vi "SngJntArmSim_Execute.vi"(5 "SngJntArmSim_Model _Params":T2={"DCMOTOR_TYPES"=enum."NEO", "Num Motors"=1, "ArmLength_M"=0.75, "massKg"=26.0, "Gearing"=128.0, "MOI kgm2"=26.0, "Estimate MOI"=TRUE} {"MOI kgm2" format="%#_13g"; "Gearing" format="%#_13g"; "massKg" format="%#_13g"; "ArmLength_M" format="%#_13g"}, 7 "SngJntArmSim_Simulation _Params":T1={"MinAngle_Rad"=0.0, "MaxAngle_Rad"=0.0, "Measurment StdDev"=0.09, "SimulateGravity"=TRUE} {"Measurment StdDev" format="%#_13g"}, 8 "dT_Seconds":dbl=0.02 format="%#_13g", 9 "Battery Volts":dbl=12.0, 11 "Motor Dmd":dbl) -> (0 "Error":bool, 1 "AtLowLimit":bool, 2 "At HIgh LImit":bool, 3 "ArmAngle_Rad":dbl, 4 "Motor Current":dbl, 6 "SingleJointArmSim":T4 {"GearBox"."Jr_KgM2" format="%13.5p"; "GearBox"."L_H" format="%13.5p"; "GearBox"."Kt_NMPerAmp" format="%13.5p"; "GearBox"."KvINV_RadPerSecPerVolt" format="%13.5p"; "GearBox"."R_Ohms" format="%13.5p"; "GearBox"."FreeSpeed_RadPerSec" format="%13.5p"; "GearBox"."FreeCurrent_Amps" format="%13.5p"; "GearBox"."StallCurrent_Amps" format="%13.5p"; "GearBox"."StallTorque_NM" format="%13.5p"; "GearBox"."nominalVoltage_Volts" format="%13.5p"})   [LabVIEW 2019, in "Trajectory_Library.lvlib"]
doc: "The single jointed arm linear system definition is:\n - States\n - angle position (Rad)\n - Inputs:\n - motor voltage\n - Outputs:\n - angle position (rad)"
uses:
  Trajectory_Library.lvlib
  TypeDef/SINGLE_JOINT_ARM_SIM.ctl
  TypeDef/LINEAR_SYSTEM_SIM.ctl
  TypeDef/LINEAR_SYSTEM.ctl
  <vilib>/Analysis/Matrix/Datatypes/RealMatrix.ctl
  TypeDef/DCMOTOR.CTL
  TypeDef/LINEAR_SYSTEM_ID_SINGLE_JOINT_ARM_MODEL.ctl
  Enum/DCMOTOR_TYPES_ENUM.ctl
  TypeDef/SINGLE_JOINT_ARM_SIM_SIMULATION_PARAMS.ctl
  MatBuilder_Create.vi
  DCMotor_GetCIM.vi
  DCMotor_GetAndymark9015.vi
  DCMotor_GetAndymarkRs775_125.vi
  DCMotor_GetBag.vi
  DCMotor_GetBanebotsRs550.vi
  DCMotor_GetBanebotsRs775.vi
  DCMotor_GetFalcon500.vi
  DCMotor_GetMiniCIM.vi
  DCMotor_GetNEO.vi
  DCMotor_GetNEO550.vi
  DCMotor_GetRomiBuiltIn.vi
  DCMotor_GetVex775Pro.vi
  DCMotor_GetAndymarkAM2235A.vi
  DCMotor_GetAndymarkAM3493.vi
  DCMotor_New.vi
  Units_RotationsPerMinuteToRadiansPerSecond.vi
  <vilib>/Analysis/Matrix/NI_Matrix.lvlib
panel:
  out "Velocity_RadsPerSec":dbl
  # "<States, 1>"
  # "<Outputs, 1>"
  # "<Inputs, 1>"
  # "<Outputs, 1>"
  # "<States,States>"
  # "<States,Inputs>"
  # "<Outputs,States>"
  # "<Outputs,Inputs>"
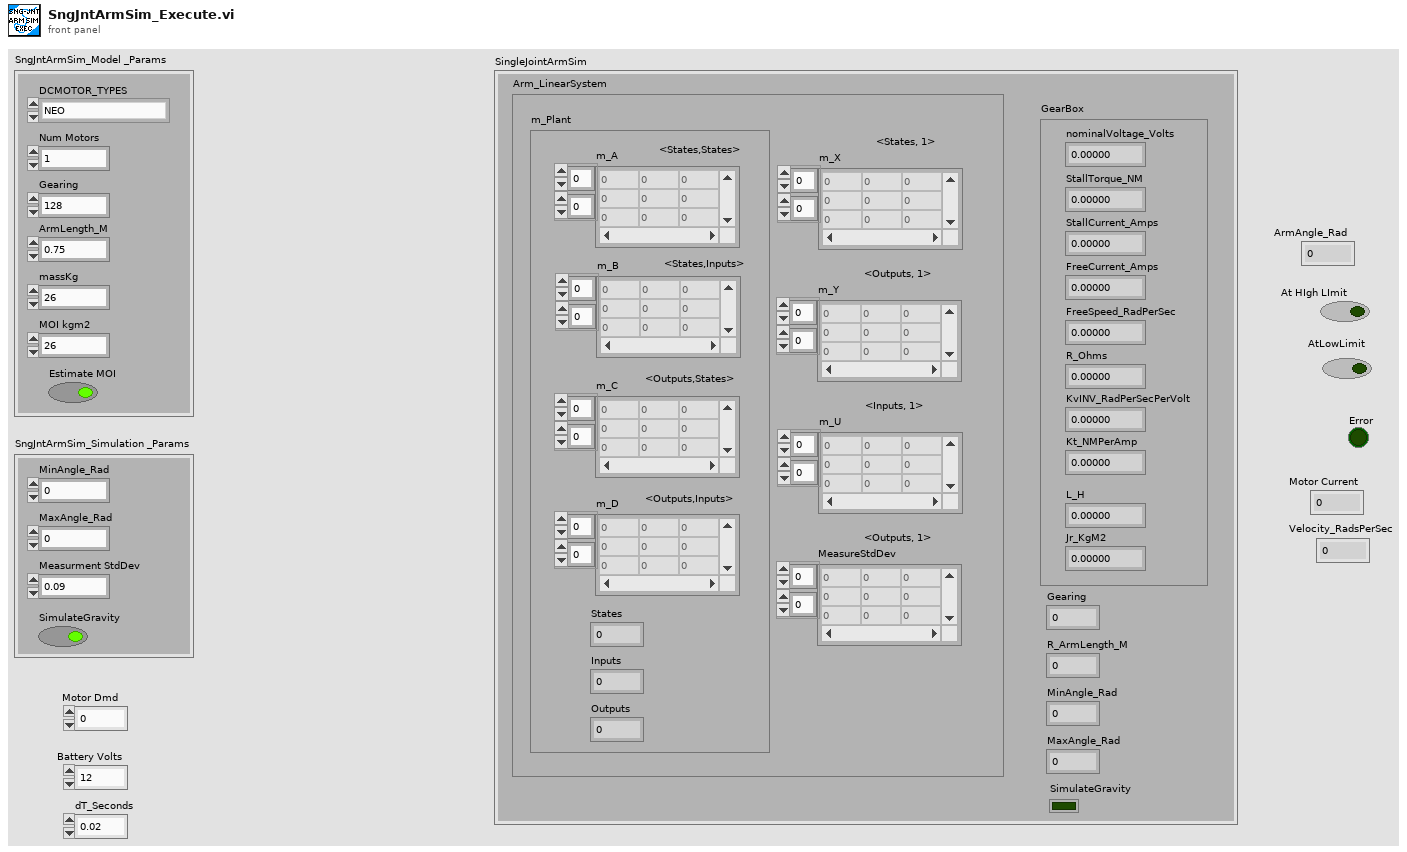
[diagram p1: front panel]
types:
  T1 = typedef "Trajectory_Library.lvlib/SINGLE_JOINT_ARM_SIM_SIMULATION_PARAMS.ctl" = cluster{"MinAngle_Rad":dbl, "MaxAngle_Rad":dbl, "Measurment StdDev":dbl, "SimulateGravity":bool}
  T2 = typedef "Trajectory_Library.lvlib/LINEAR_SYSTEM_ID_SINGLE_JOINT_ARM_MODEL.ctl" = cluster{"DCMOTOR_TYPES":T3, "Num Motors":i32, "ArmLength_M":dbl, "massKg":dbl, "Gearing":dbl, "MOI kgm2":dbl, "Estimate MOI":bool}
  T3 = typedef "Trajectory_Library.lvlib/DCMOTOR_TYPES_ENUM.ctl" = enum16{"CIM", "AndyMark 9015", "Andy Mark RS 775 125", "Bag", "BaneBots RS 550", "BaneBots RS 775", "Falcon 500", "Mini CIM", "NEO", "NEO 550", "Romi BuiltIn", "Vex 775 Pro", "Snow Blower AM 2235A", "Bosch Seat AM 3493"}
  T4 = typedef "Trajectory_Library.lvlib/SINGLE_JOINT_ARM_SIM.ctl" = cluster{"Arm_LinearSystem":T5, "GearBox":T8, "Gearing":dbl, "R_ArmLength_M":dbl, "MinAngle_Rad":dbl, "MaxAngle_Rad":dbl, "SimulateGravity":bool}
  T5 = typedef "Trajectory_Library.lvlib/LINEAR_SYSTEM_SIM.ctl" = cluster{"m_Plant":T6, "m_X":T7, "m_Y":T7, "m_U":T7, "MeasureStdDev":T7}
  T6 = typedef "Trajectory_Library.lvlib/LINEAR_SYSTEM.ctl" = cluster{"m_A":T7, "m_B":T7, "m_C":T7, "m_D":T7, "States":i32, "Inputs":i32, "Outputs":i32}
  T7 = typedef "NI_Matrix.lvlib/RealMatrix.ctl" = dbl[][]
  T8 = typedef "Trajectory_Library.lvlib/DCMOTOR.CTL" = cluster{"nominalVoltage_Volts":dbl, "StallTorque_NM":dbl, "StallCurrent_Amps":dbl, "FreeCurrent_Amps":dbl, "FreeSpeed_RadPerSec":dbl, "R_Ohms":dbl, "KvINV_RadPerSecPerVolt":dbl, "Kt_NMPerAmp":dbl, "L_H":dbl, "Jr_KgM2":dbl}
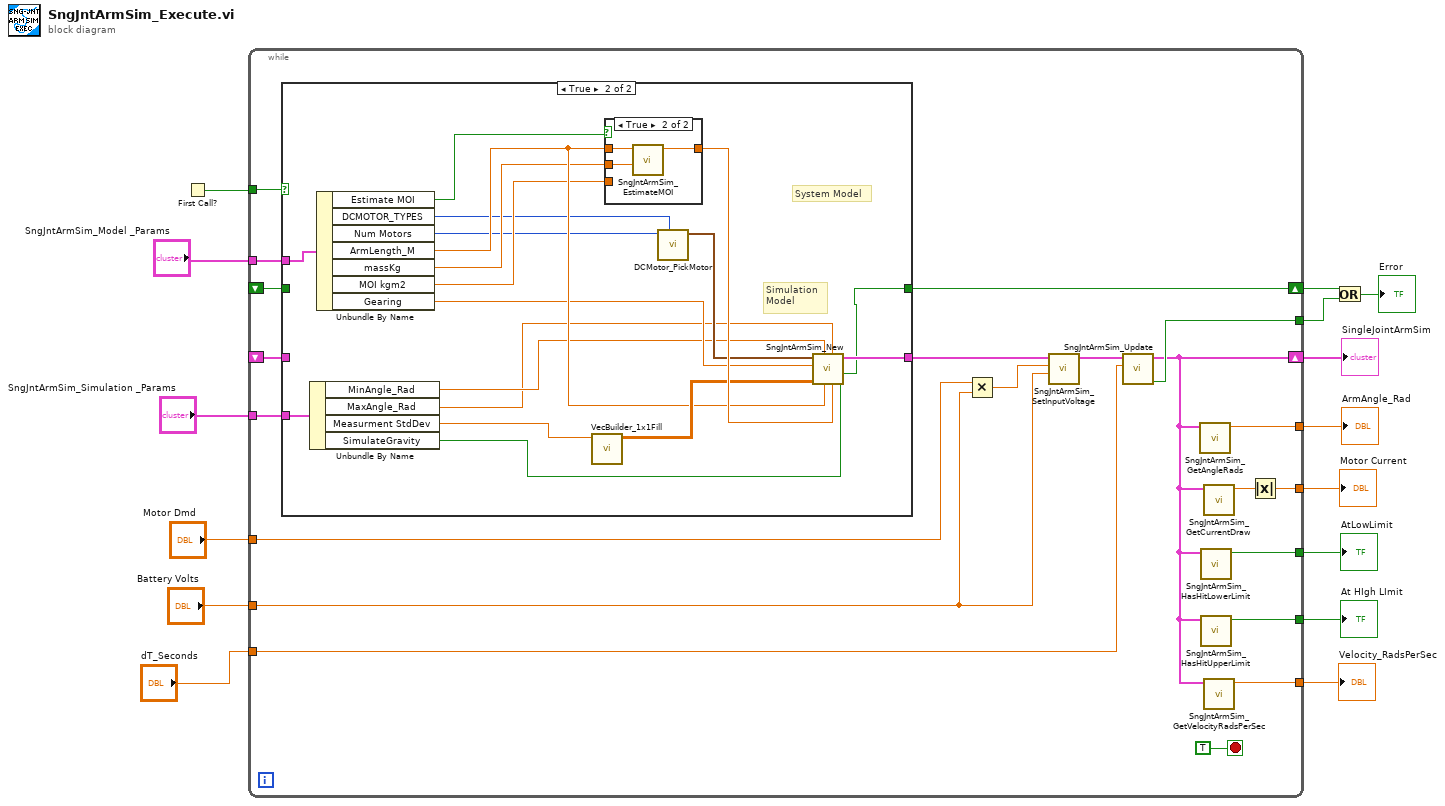
[diagram p0: block diagram]
diagram:
  n1 = First Call?() -> (First Call?: T/F=w13:bool)
  n2 = while {
    tunnel: "SngJntArmSim_Model _Params" -> [w36]
    tunnel: w13 -> [w35]
    shift-right: [w17] -> w15
    shift-left: _ -> [w34]
    shift-right: [w33] -> w6
    shift-left: _ -> [w32]
    tunnel: "Motor Dmd" -> [w27]
    tunnel: "Battery Volts" -> [w26]
    tunnel: [w25] -> w10
    tunnel: [w23] -> w9
    tunnel: [w22] -> w8
    tunnel: [w21] -> w7
    tunnel: [w20] -> w5
    tunnel: "dT_Seconds" -> [w19]
    tunnel: "SngJntArmSim_Simulation _Params" -> [w18]
    tunnel: [w16] -> w1
    stop <- TRUE stop-if-true
    n3 = case shown="True" w35 {
      tunnel: [w38 w53] -> w28
      tunnel: w36 -> [_ w52]
      tunnel: w34 -> [w38 _]
      tunnel: [w37 w39] -> w33
      tunnel: w32 -> [w37 _]
      tunnel: w18 -> [_ w44]
      frame False {
      }
      frame True {
        # "Simulation \nModel"
        # "System Model"
        n4 = Unbundle By Name(w44) -> ("MinAngle_Rad"=w41:dbl, "MaxAngle_Rad"=w40:dbl, "Measurment StdDev"=w43:dbl, "SimulateGravity"=w42:bool)
        n5 = Unbundle By Name(w52) -> ("Estimate MOI"=w45:bool, "DCMOTOR_TYPES"=w46:T3, "Num Motors"=w47:i32, "ArmLength_M"=w51:dbl, "massKg"=w48:dbl, "MOI kgm2"=w49:dbl, "Gearing"=w50:dbl)
        n6 = call "VecBuilder_1x1Fill.vi"("R0_C0"=w43) -> ("output matrix"=w55:T7)  [unwired: 10 in]
        n7 = case shown="True" w45 {
          tunnel: [w57 w60] -> w56
          tunnel: w48 -> [_ w59]
          tunnel: w51 -> [_ w58]
          tunnel: w49 -> [w57 _]
          frame False {
          }
          frame True {
            n8 = call "SngJntArmSim_EstimateMOI.vi"("ArmMass_Kg"=w59, "ArmLength_M"=w58) -> ("MOI"=w60:dbl)  [unwired: 9 in]
          }
        }
        n9 = call "DCMotor_PickMotor.vi"("DCMOTOR_TYPES"=w46, "Num Motors"=w47) -> ("DCMOTOR"=w54:T8)  [unwired: 9 in]
        n10 = call "SngJntArmSim_New.vi"("SimulateGravity"=w42, "jKgMetersSquared"=w56, "MaxAngle_Rad"=w40, "ArmLength_Meters"=w51, "MinAngle_Rad"=w41, "MeasurementStdDev"=w55, "Gearing"=w50, "GearBox"=w54) -> ("Error"=w39:bool, "SingleJointArmSim"=w53:T4)  [unwired: 2 in]
      }
    }
    n11 = Multiply(x=w27, y=w26) -> (x*y=w31:dbl)
    n12 = call "SngJntArmSim_SetInputVoltage.vi"("Battery_Volts"=w26, "Input_Voltage"=w31, "in SingleJointArmSim"=w28) -> ("out SingleJointArmSim"=w29:T4)  [unwired: 8 in]
    n13 = call "SngJntArmSim_Update.vi"("dT_Seconds"=w19, "in SingleJointArmSim"=w29) -> ("Error"=w20:bool, "out SingleJointArmSim"=w17:T4)  [unwired: 8 in]
    n14 = call "SngJntArmSim_GetAngleRads.vi"("SingleJointArmSim"=w17) -> ("ArmAngle_Rad"=w23:dbl)  [unwired: 10 in]
    n15 = call "SngJntArmSim_HasHitLowerLimit.vi"("SingleJointArmSim"=w17) -> ("AtLowLimit"=w21:bool)  [unwired: 10 in]
    n16 = call "SngJntArmSim_HasHitUpperLimit.vi"("SingleJointArmSim"=w17) -> ("At HIgh LImit"=w22:bool)  [unwired: 10 in]
    n17 = call "SngJntArmSim_GetCurrentDraw.vi"("SingleJointArmSim"=w17) -> ("Current_Amps"=w30:dbl)  [unwired: 10 in]
    n18 = call "SngJntArmSim_GetVelocityRadsPerSec.vi"("singleJointArmSim"=w17) -> ("Velocity_RadsPerSec"=w16:dbl)  [unwired: 10 in]
    n19 = Absolute Value(x=w30) -> (abs(x)=w25:dbl)
  }
  "SingleJointArmSim" <- w15
  "Motor Current" <- w10
  "ArmAngle_Rad" <- w9
  "AtLowLimit" <- w7
  "At HIgh LImit" <- w8
  "Velocity_RadsPerSec" <- w1
  n20 = Or(x=w6, y=w5) -> (x .or. y?=→"Error":bool)
